vi "运维调试_HACH多参.vi"() -> ()   [LabVIEW 2016, in "HACH多参.lvlib"]
uses:
  <vilib>/Utility/miscctls.llb/LVPointTypeDef.ctl
  <vilib>/Plasmionique/MB Master/MB_ADU/MB_ADU.lvclass/MB_ADU.ctl
  <vilib>/Plasmionique/MB Master/MB_ADU/Read TX Timestamp.vi
  <vilib>/Plasmionique/MB Master/MB_ADU/Read TX Data.vi
  <vilib>/Plasmionique/MB Master/MB_ADU/Read RX Timestamp.vi
  <vilib>/Plasmionique/MB Master/MB_ADU/Read RX Data.vi
  <vilib>/Plasmionique/MB Master/MB_Master_Serial/MB_Master_Serial.lvclass
  F:/Program Files/National Instruments/LabVIEW 2016/vi.lib/Plasmionique/MB Master/MB_Master/MB_Master.lvclass
  <vilib>/Plasmionique/MB Master/MB_ADU/MB_ADU.lvclass
  <vilib>/Plasmionique/MB Master/MB Master.lvlib
panel:
  in  "停止":bool
  out "运行状态":string
  in  "水样测试":bool
  in  "返回":bool
  in  "设置":bool
  out "LOG":string
  out "小项目框 8":T1(xcontrol)
  out "小项目框 7":T1(xcontrol)
  out "小项目框 6":T1(xcontrol)
  out "小项目框 5":T1(xcontrol)
  out "小项目框 4":T1(xcontrol)
  out "小项目框 3":T1(xcontrol)
  out "小项目框 2":T1(xcontrol)
  out "小项目框":T1(xcontrol)
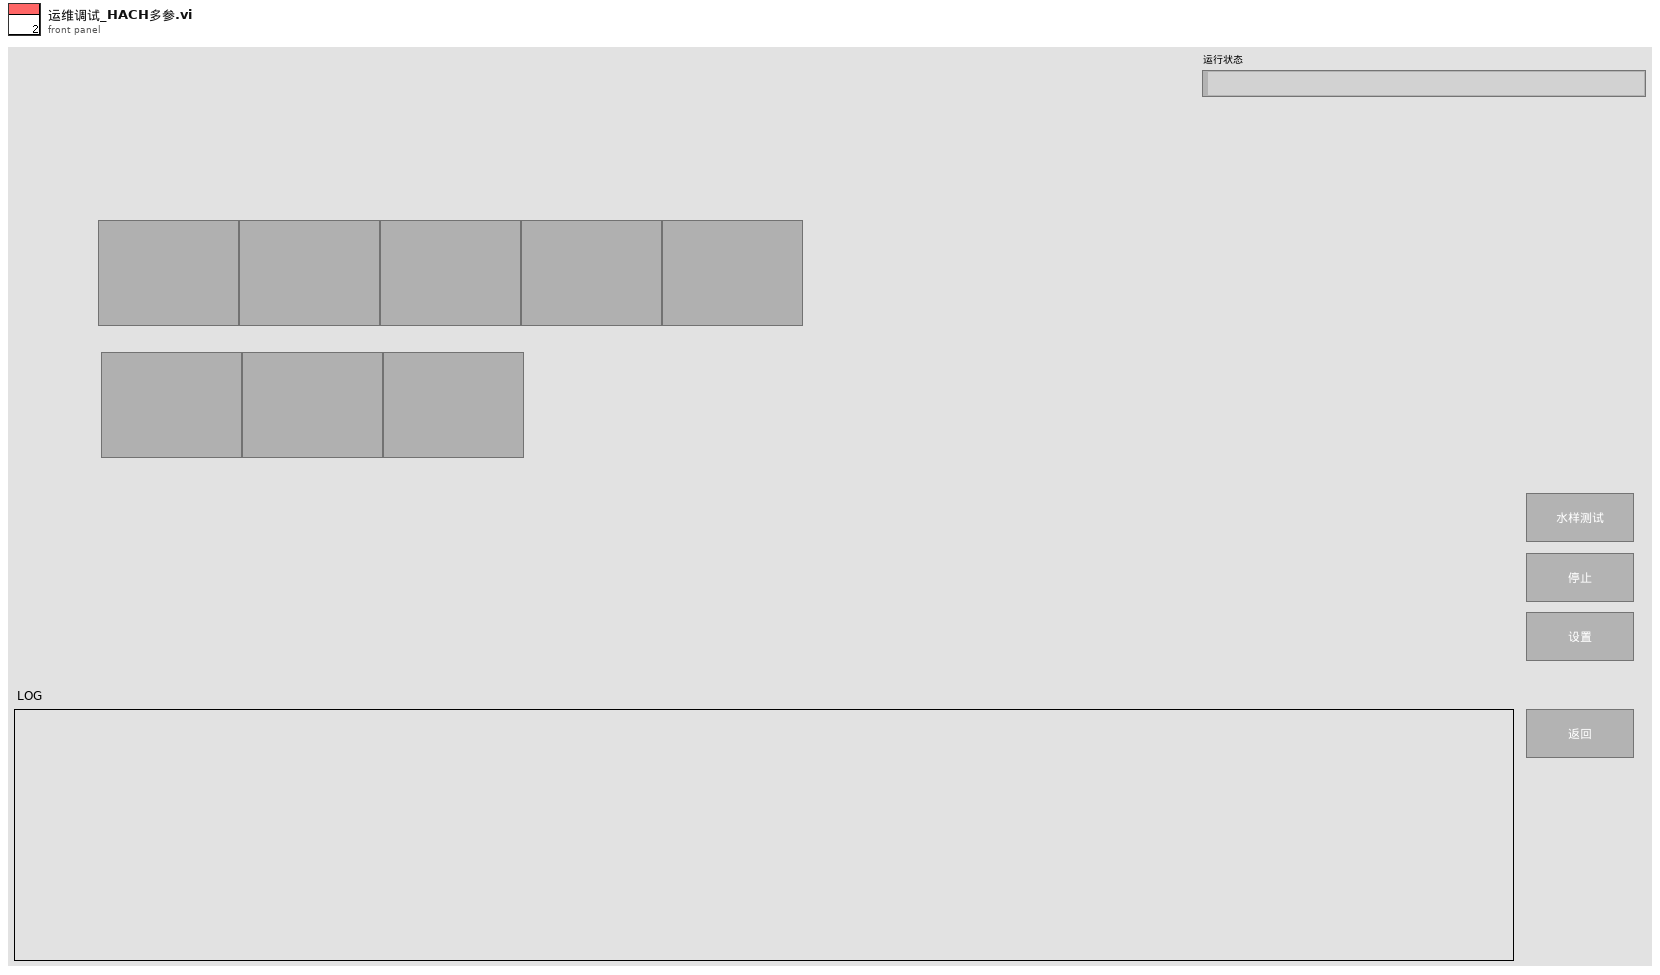
[diagram p1: front panel]
types:
  T1 = cluster{"中文项目名称":string, "英文项目名称":string, "单位":string, "浓度值":sgl, "精度":sgl}
  T2 = typedef "LVPointTypeDef.ctl" = cluster{"Horizontal":i16, "Vertical":i16}
  T3 = cluster{"DO_Temp":dbl, "DO_mg/L":dbl, "DO_%":dbl, "pH_Temp":dbl, "pH":dbl, "Turb":dbl, "Cond_Temp":dbl, "Cond":dbl, "Sat":dbl}
  T4 = cluster{"测试时间":dbl, "运行模式":enum16{"维护模式", "常规模式", "应急模式", "质控模式"}}
  T5 = enum32{"Bad", "Idle", "Run top level", "Running"}
  T6 = cluster{"baud rate (bps)":u32, "stop bits":u16, "parity":u16, "flow control":u16, "timeout":u32, "retries":i32}
  T7 = cluster{"[0]":sgl, "[1]":sgl, "[2]":sgl, "[3]":sgl, "[4]":sgl, "[5]":sgl, "[6]":sgl, "[7]":sgl, "[8]":sgl}
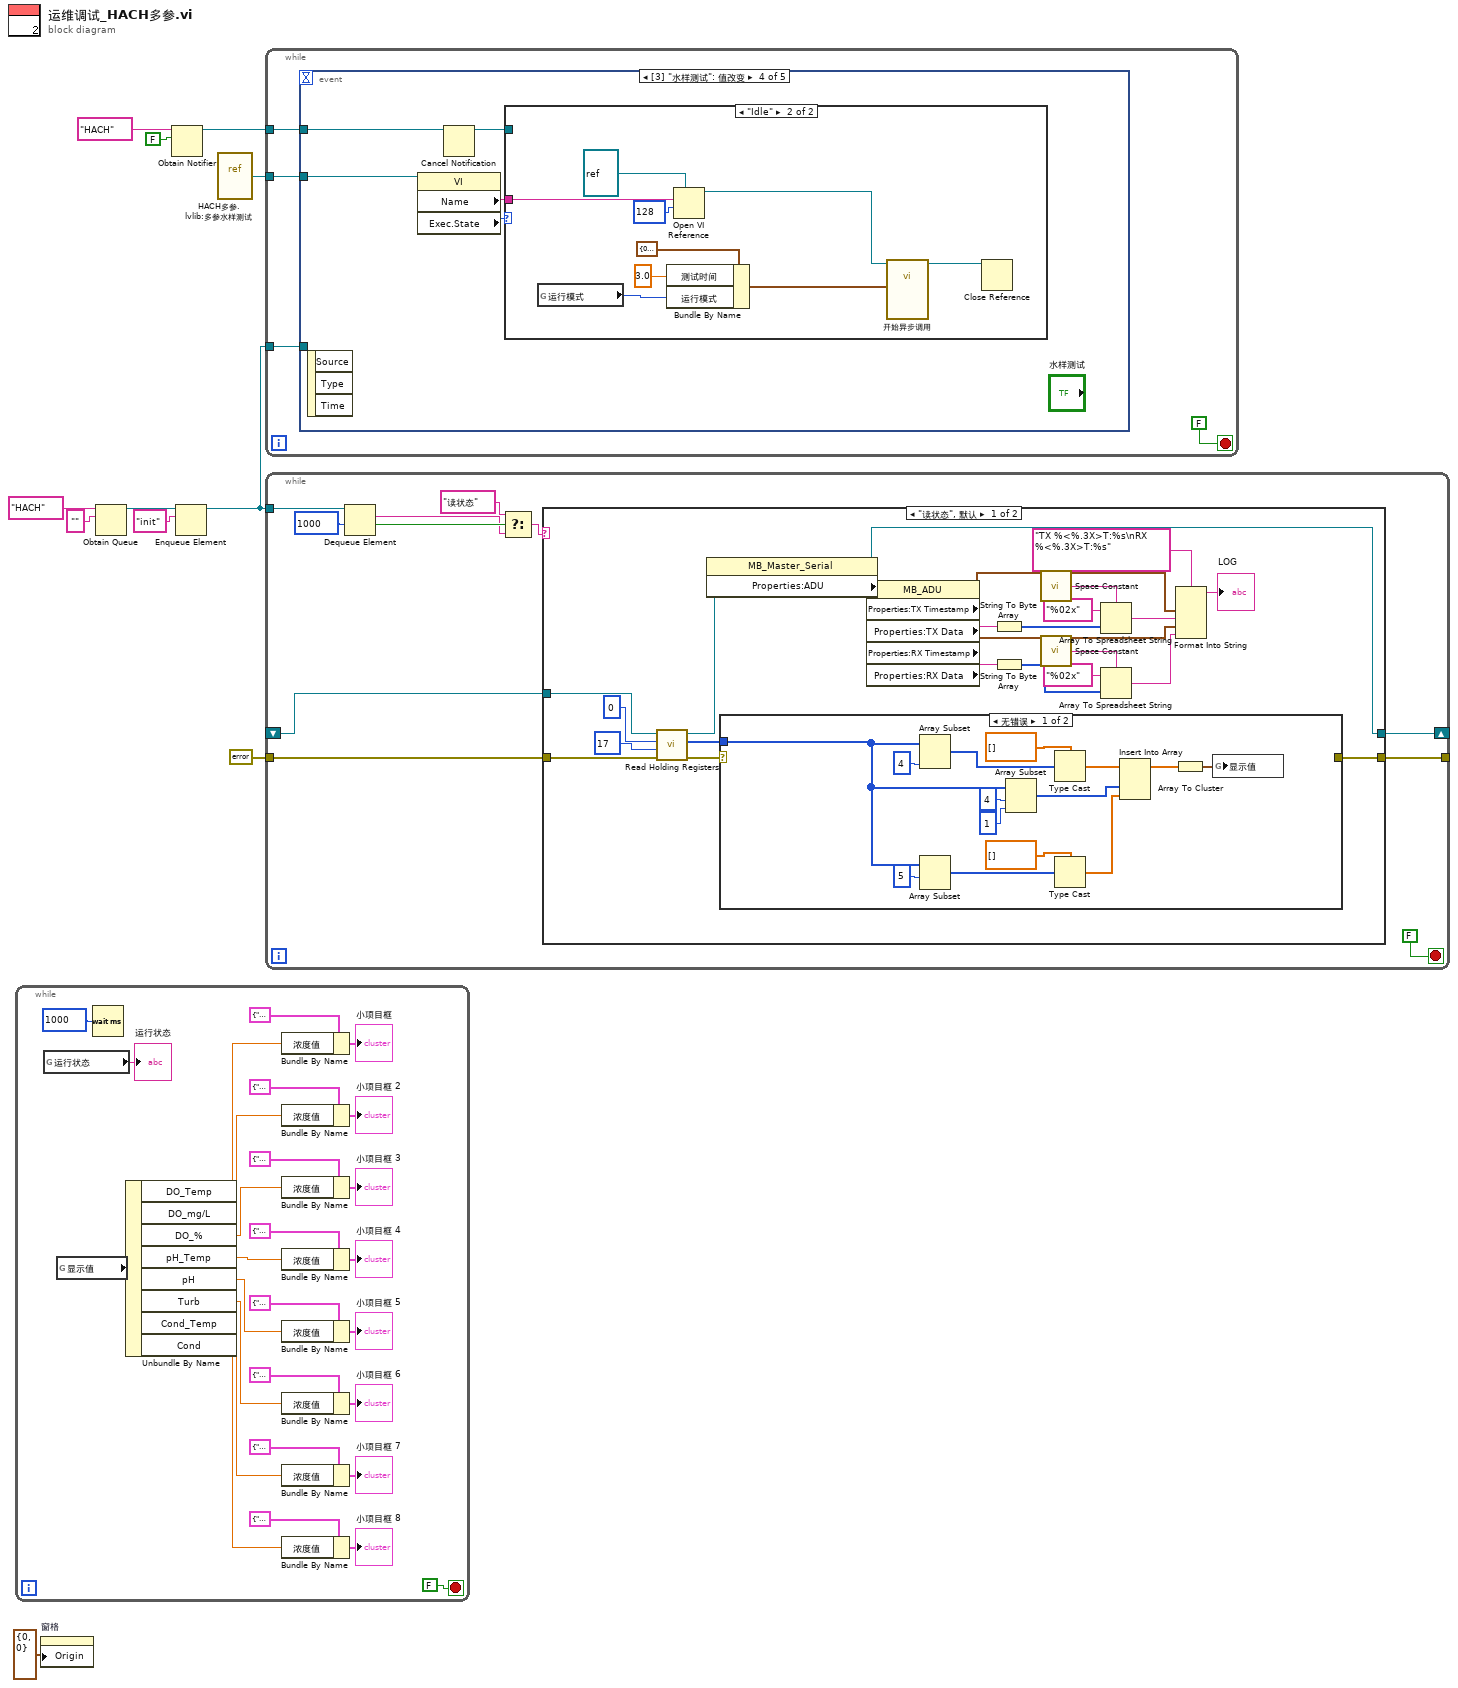
[diagram p0: block diagram]
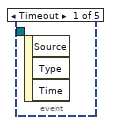
[diagram p2: hidden frame]
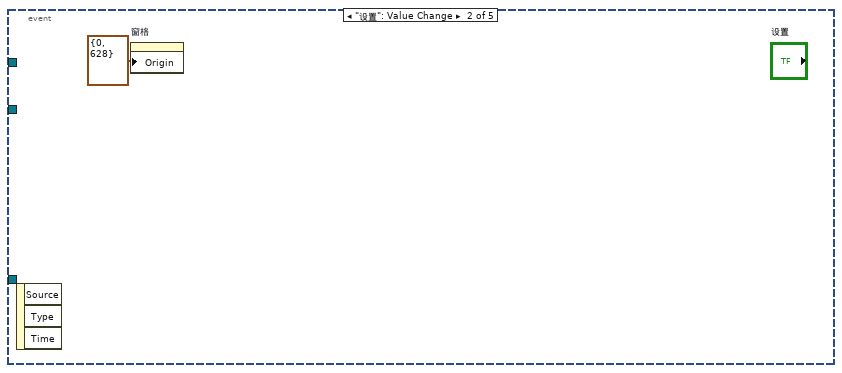
[diagram p3: hidden frame]
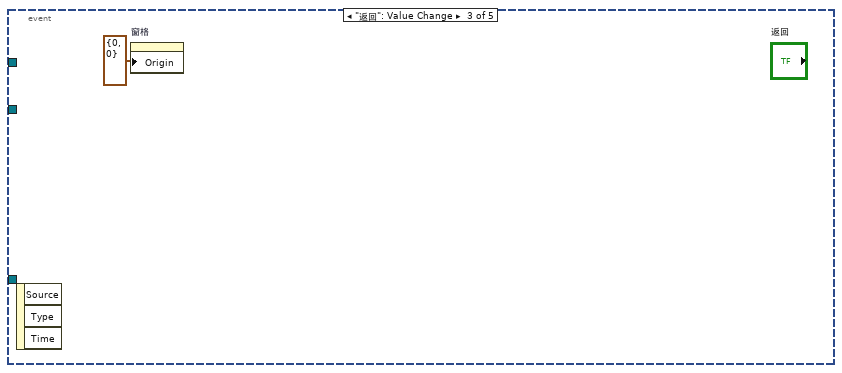
[diagram p4: hidden frame]
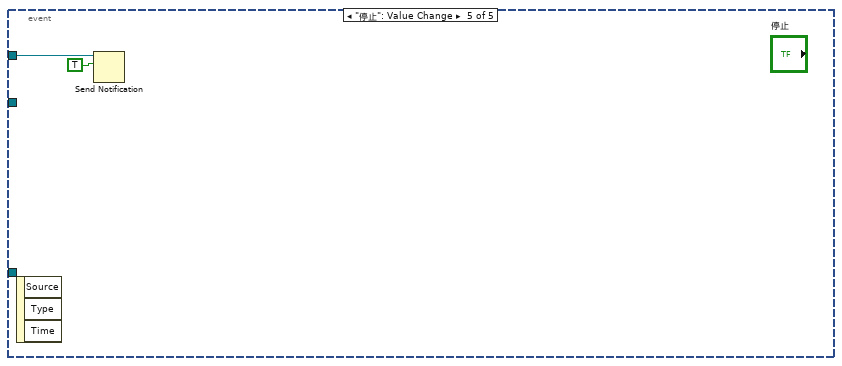
[diagram p6: hidden frame]
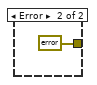
[diagram p7: hidden frame]
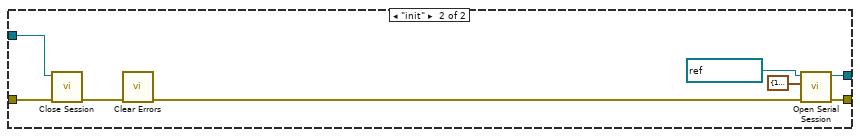
[diagram p8: hidden frame]
diagram:
  n1 = while {
    stop <- FALSE stop-if-true
    n2 = global read "HACH全局.vi" "运行状态"() -> (→"运行状态":string)
    n3 = global read "HACH全局.vi" "显示值"() -> (w37:T3)
    n4 = Wait (ms)(milliseconds to wait=u32 1000 ("等待时间（毫秒）")) -> ()  [unwired: 1 out]
    n5 = Unbundle By Name(w37) -> ("DO_Temp"=w34:dbl, "DO_mg/L"=w33:dbl, "DO_%"=w29:dbl, "pH_Temp"=w26:dbl, "pH"=w23:dbl, "Turb"=w19:dbl, "Cond_Temp"=w16:dbl, "Cond"=w13:dbl)
    n6 = Bundle By Name(cluster=T1 {"中文项目名称"="溶解氧温度", "英文项目名称"="DO_Temp", "单位"="℃", "浓度值"=0.0, "精度"=2.0} ("小项目框"), "浓度值"=w34) -> (→"小项目框":T1)
    n7 = Bundle By Name(cluster=T1 {"中文项目名称"="溶解氧", "英文项目名称"="DO", "单位"="mg/L", "浓度值"=0.0, "精度"=2.0} ("小项目框"), "浓度值"=w33) -> (→"小项目框 2":T1)
    n8 = Bundle By Name(cluster=T1 {"中文项目名称"="溶解氧", "英文项目名称"="DO", "单位"="%", "浓度值"=0.0, "精度"=2.0} ("小项目框"), "浓度值"=w29) -> (→"小项目框 3":T1)
    n9 = Bundle By Name(cluster=T1 {"中文项目名称"="酸碱度温度", "英文项目名称"="pH_Temp", "单位"="℃", "浓度值"=0.0, "精度"=2.0} ("小项目框"), "浓度值"=w26) -> (→"小项目框 4":T1)
    n10 = Bundle By Name(cluster=T1 {"中文项目名称"="酸碱度", "英文项目名称"="pH", "单位"="", "浓度值"=0.0, "精度"=2.0} ("小项目框"), "浓度值"=w23) -> (→"小项目框 5":T1)
    n11 = Bundle By Name(cluster=T1 {"中文项目名称"="浊度", "英文项目名称"="Turb", "单位"="NTU", "浓度值"=0.0, "精度"=2.0} ("小项目框"), "浓度值"=w19) -> (→"小项目框 6":T1)
    n12 = Bundle By Name(cluster=T1 {"中文项目名称"="电导率温度", "英文项目名称"="Cond_Temp", "单位"="℃", "浓度值"=0.0, "精度"=2.0} ("小项目框"), "浓度值"=w16) -> (→"小项目框 7":T1)
    n13 = Bundle By Name(cluster=T1 {"中文项目名称"="电导率", "英文项目名称"="Cond", "单位"="ms/cm", "浓度值"=0.0, "精度"=2.0} ("小项目框"), "浓度值"=w13) -> (→"小项目框 8":T1)
  }
  n14 = property on="窗格" class="Pane"("Origin"=T2 {"Horizontal"=0, "Vertical"=0} ("原点")) -> ()  [unwired: 2 in, 2 out]
  n15 = Obtain Queue(name (unnamed)="HACH" ("名称（未命名）"), element data type="") -> (queue out=w8:refnum<queue>)  [unwired: 3 in, 2 out]
  n16 = Obtain Notifier(name (unnamed)="HACH" ("名称（未命名）"), notification data type=FALSE) -> (notifier out=w2:refnum<notifier>)  [unwired: 2 in, 2 out]
  n17 = Enqueue Element(queue=w8, element="init" ("元素")) -> (queue out=w7:refnum<queue>)  [unwired: 2 in, 2 out]
  n18 = vi-ref "HACH多参.lvlib:多参水样测试.vi"() -> (w4:refnum<vi>)
  n19 = while {
    tunnel: w7 -> [w42]
    tunnel: w4 -> [w41]
    tunnel: w2 -> [w40]
    stop <- FALSE stop-if-true
    n20 = event shown="[3] \"水样测试\": 值改变" {
      selector: _ -> [_ _ _ _ _]
      dyn-events: _ -> [_ _ _ _ _]
      timeout: _ -> [_ _ _ _ _]
      tunnel: w42 -> [_ _ _ _ _]
      tunnel: w41 -> [_ _ _ w50 _]
      tunnel: w40 -> [_ _ _ w47 w61]
      event Timeout {
        n21 = event-data() -> ()  [unwired: 1 in, 3 out]
      }
      event "设置": Value Change {
        n22 = event-data() -> ()  [unwired: 1 in, 3 out]
        n23 = property on="窗格" class="Pane"("Origin"=T2 {"Horizontal"=0, "Vertical"=628} ("原点")) -> ()  [unwired: 2 in, 2 out]
      }
      event "返回": Value Change {
        n24 = event-data() -> ()  [unwired: 1 in, 3 out]
        n25 = property on="窗格" class="Pane"("Origin"=T2 {"Horizontal"=0, "Vertical"=0} ("原点")) -> ()  [unwired: 2 in, 2 out]
      }
      event "水样测试": Value Change {
        n26 = event-data() -> ()  [unwired: 1 in, 3 out]
        n27 = property class="VI"(reference=w50) -> ("Name"=w49:string, "Exec.State"=w48:T5)  [unwired: 1 in, 2 out]
        n28 = Cancel Notification(0:w47) -> (8:w46:refnum<notifier>)  [unwired: 1 in, 2 out]
        n29 = case shown="\"Idle\"" w48 {
          tunnel: w49 -> [_ w59]
          tunnel: w46 -> [_ _]
          frame "Bad", Default {
          }
          frame "Idle" {
            n30 = global read "系统变量.vi" "运行模式"() -> (w51:enum16{"维护模式", "常规模式", "应急模式", "质控模式"})
            n31 = Bundle By Name(cluster=T4 {"测试时间"=0.0, "运行模式"=enum."维护模式"} ("API"), "测试时间"=3.0, "运行模式"=w51) -> (w55:T4)
            n32 = Open VI Reference(type specifier VI Refnum (for type only)=refnum<vi> refnum ("类型说明符VI引用句柄（仅用于类型）"), vi path=w59, options=128 ("选项")) -> (vi reference=w53:refnum<vi>)  [unwired: 3 in, 1 out]
            n33 = call-by-ref "开始异步调用"(reference=w53, "API"=w55) -> (reference out=w52:refnum<vi>)  [unwired: 12 in, 1 out]
            n34 = Close Reference(reference=w52) -> ()  [unwired: 1 in, 1 out]
          }
        }
      }
      event "停止": Value Change {
        n35 = event-data() -> ()  [unwired: 1 in, 3 out]
        n36 = Send Notification(notification=TRUE ("通知"), notifier=w61) -> ()  [unwired: 1 in, 2 out]
      }
    }
  }
  n37 = while {
    tunnel: [w71] -> _
    shift-right: [w72] -> _
    shift-left: _ -> [w70]
    tunnel: errorcluster {"status"=FALSE, "code"=0, "source"=""} ("error in (no error)") -> [w69]
    tunnel: w7 -> [w68]
    stop <- FALSE stop-if-true
    n38 = Dequeue Element(queue=w68, timeout in ms (-1)=1000 ("超时毫秒(-1)")) -> (element=w64:string, timed out?=w66:bool)  [unwired: 1 in, 2 out]
    n39 = Select(t="读状态" ("元素"), s=w66, f=w64) -> (s? t:f=w63:string)
    n40 = case shown="\"读状态\", 默认" w63 {
      tunnel: [w88 w119] -> w72
      tunnel: [w90 w118] -> w71
      tunnel: w70 -> [w96 w117]
      tunnel: w69 -> [w95 w116]
      frame "读状态", Default {
        n41 = call <vilib>:"Read Holding Registers.vi"("error in (no error)"=w95, "quantity"=u16 17, "starting address"=u16 0, "MB session in"=w96) -> ("error out"=w91:errorcluster, "Registers"=w92:u16[], "MB session out"=w89:refnum<class "MB_Master_Serial.lvclass">)  [unwired: 5 in]
        n42 = property class="MB_Master_Serial"(reference=w89) -> (reference out=w88:refnum<class "MB_Master_Serial.lvclass">, "Properties:ADU"=w87:refnum<class "MB_ADU.lvclass">)  [unwired: 1 in, 1 out]
        n43 = case shown="无错误" w91 {
          tunnel: w92 -> [w105 _]
          tunnel: [_ errorcluster {"status"=FALSE, "code"=0, "source"=""} ("error IO")] -> w90
          frame No Error {
            n44 = Array Subset(array=w105, length=4 ("长度")) -> (w108:u16[])  [unwired: 1 in]
            n45 = Array Subset(array=w105, index=5 ("索引")) -> (w103:u16[])  [unwired: 1 in]
            n46 = Array Subset(array=w105, index=4 ("索引"), length=1 ("长度")) -> (w100:u16[])
            n47 = Type Cast(type=sgl[] [], x=w108) -> (*(type *) &x=w101:sgl[])
            n48 = Type Cast(type=sgl[] [], x=w103) -> (*(type *) &x=w99:sgl[])
            n49 = Insert Into Array(array=w101, new element #1=w100, new element #2=w99) -> (w98:sgl[])  [unwired: 1 in]
            n50 = Array To Cluster(array=w98) -> (cluster=w97:T7)
            n51 = global write "HACH全局.vi" "显示值"(w97) -> ()
          }
          frame Error {
          }
        }
        n52 = property class="MB_ADU"(reference=w87) -> ("Properties:TX Timestamp"=w86:timestamp, "Properties:TX Data"=w79:string, "Properties:RX Timestamp"=w85:timestamp, "Properties:RX Data"=w75:string)  [unwired: 1 in, 2 out]
        n53 = String To Byte Array(string=w79) -> (unsigned byte array=w81:u8[])
        n54 = String To Byte Array(string=w75) -> (unsigned byte array=w77:u8[])
        n55 = call <vilib>:"Space Constant.vi"() -> ("String"=w82:string)
        n56 = call <vilib>:"Space Constant.vi"() -> ("String"=w78:string)
        n57 = Array To Spreadsheet String(delimiter (Tab)=w82, array=w81, 3:"%02x" ("格式字符串")) -> (spreadsheet string=w73:string)
        n58 = Array To Spreadsheet String(delimiter (Tab)=w78, array=w77, 3:"%02x" ("格式字符串")) -> (spreadsheet string=w74:string)
        n59 = Format Into String(format string="TX %<%.3X>T:%s\nRX %<%.3X>T:%s" ("格式字符串"), w86, w73, w85, w74) -> (resulting string=→"LOG":string)  [unwired: 2 in, 1 out]
      }
      frame "init" {
        n60 = call-dynamic "Close Session.vi"("error in (no error)"=w116, "MB_Serial session"=w117) -> ("error out"=w115:errorcluster)  [unwired: 9 in]
        n61 = call <vilib>:"Clear Errors.vi"("error in (no error)"=w115) -> ("error out"=w114:errorcluster)  [unwired: 5 in, 1 out]
        n62 = call <vilib>:"Open Serial Session.vi"("Error in"=w114, "Serial Config"=T6 {"baud rate (bps)"=19200, "stop bits"=10, "parity"=0, "flow control"=0, "timeout"=1000, "retries"=1}, "VISA Resource"=refnum<visa-resource-name> "COM6") -> ("Error out"=w118:errorcluster, "MB_Serial session"=w119:refnum<class "MB_Master_Serial.lvclass">)  [unwired: 7 in]
      }
    }
  }
